vi "Transfer LLP Packets To Host.vi"(0 "tagged llp packets cluster":T1, 1 "reset":bool, 5 "end of data":bool[](array[boolean])=[FALSE, FALSE, FALSE, FALSE, FALSE, FALSE, FALSE, FALSE], 9 "tagged llp packet valid":bool[](array[boolean])=[FALSE, FALSE, FALSE, FALSE, FALSE, FALSE, FALSE, FALSE]) -> (14 "ready for input":bool[](array[boolean]))   [LabVIEW 2020, in "GettingStarted_Acq_Tap_148X_FPGA.lvlib"]
uses:
  GettingStarted_Acq_Tap_148X_FPGA.lvlib
  Common/Types/Tagged LLP Packets Cluster.ctl
  <instrlib>/FlexRIO/CSI-2/v2/FPGA/Types/Tagged LLP Packet.ctl
  <instrlib>/FlexRIO/CSI-2/v2/FPGA/Types/FPGA LLP Packet Tag.ctl
  <instrlib>/FlexRIO/CSI-2/v2/FPGA/Types/FPGA LLP Packet Timestamp.ctl
  <instrlib>/FlexRIO/CSI-2/v2/FPGA/Types/Timestamp ID.ctl
  <instrlib>/FlexRIO/CSI-2/v2/FPGA/Types/FPGA LLP Packet Size.ctl
  <instrlib>/FlexRIO/CSI-2/v2/FPGA/Types/LLP Packet.ctl
  <instrlib>/FlexRIO/CSI-2/v2/FPGA/Types/LLP Packet Header.ctl
  <instrlib>/FlexRIO/CSI-2/v2/FPGA/Types/LLP Packet Payload.ctl
  <instrlib>/FlexRIO/CSI-2/v2/FPGA/Types/LLP Packet Footer.ctl
  <instrlib>/_niInstr/Basic Elements/v1/FPGA/niInstr Basic Elements v1 FPGA.lvlib
  <instrlib>/FlexRIO/CSI-2/v2/FPGA/NI CSI-2 API FPGA v2.lvlib
  Common/GettingStarted_Common_148X_FPGA.lvlib
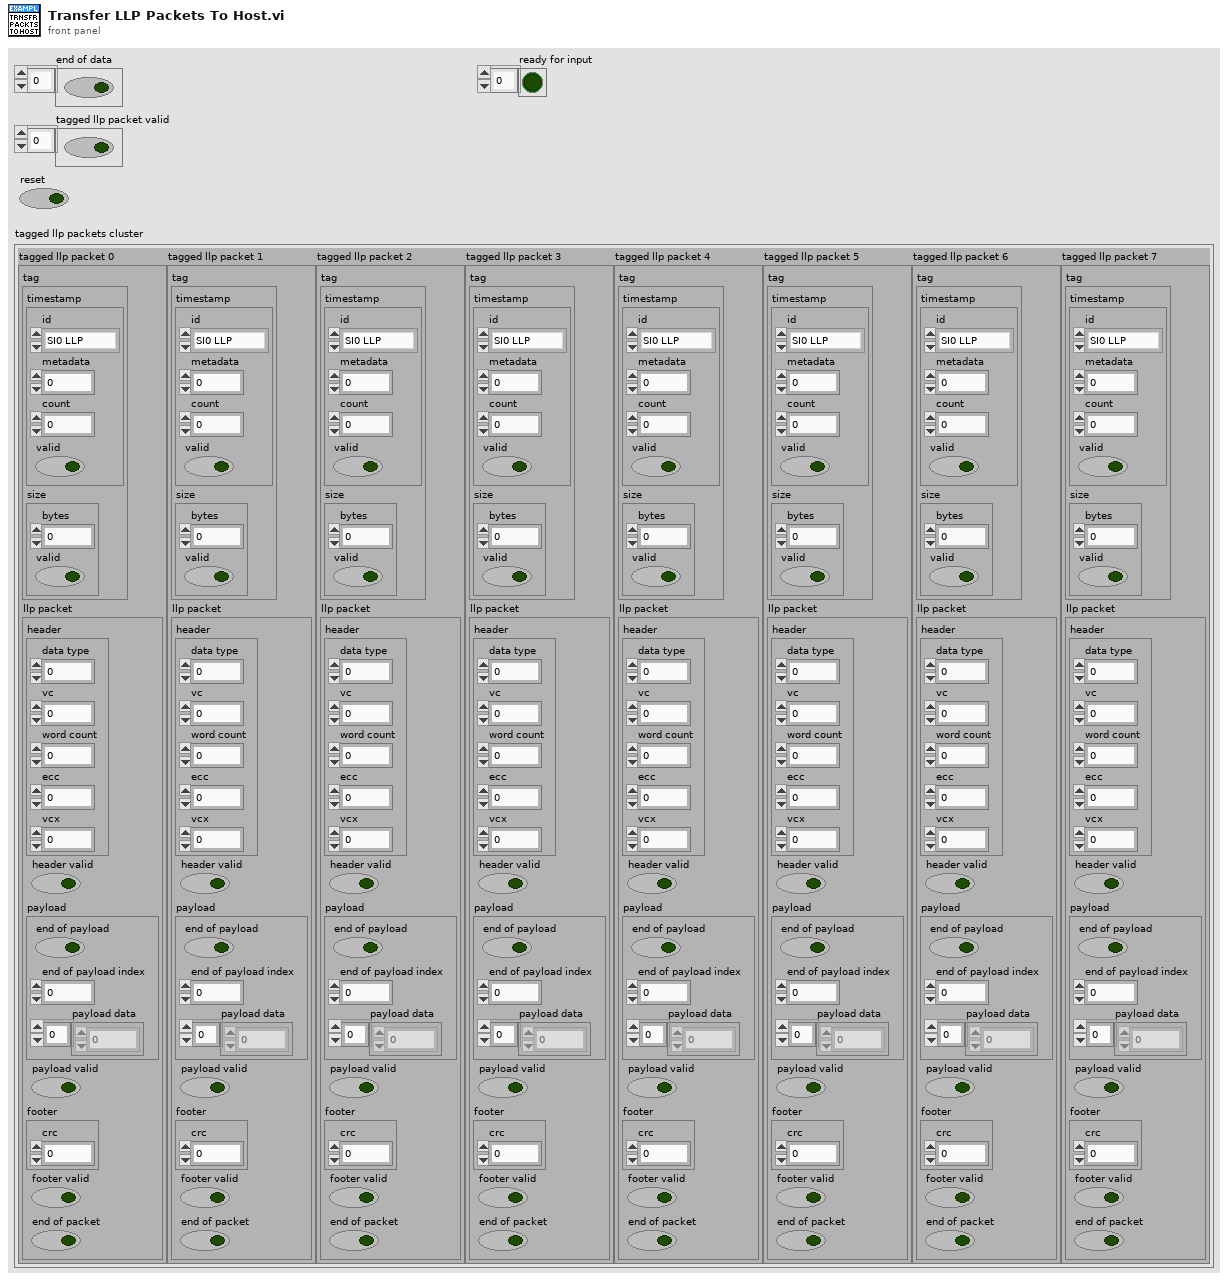
[diagram p1: front panel]
types:
  T1 = typedef "GettingStarted_Common_148X_FPGA.lvlib/Tagged LLP Packets Cluster.ctl" = cluster{"tagged llp packet 0":T2, "tagged llp packet 1":T2, "tagged llp packet 2":T2, "tagged llp packet 3":T2, "tagged llp packet 4":T2, "tagged llp packet 5":T2, "tagged llp packet 6":T2, "tagged llp packet 7":T2}
  T2 = typedef "NI CSI-2 API FPGA v2.lvlib/Tagged LLP Packet.ctl" = cluster{"tag":T3, "llp packet":T7}
  T3 = typedef "NI CSI-2 API FPGA v2.lvlib/FPGA LLP Packet Tag.ctl" = cluster{"timestamp":T4, "size":T6}
  T4 = typedef "NI CSI-2 API FPGA v2.lvlib/FPGA LLP Packet Timestamp.ctl" = cluster{"valid":bool, "count":fxp<+,50,50>, "id":T5, "metadata":u8}
  T5 = typedef "NI CSI-2 API FPGA v2.lvlib/Timestamp ID.ctl" = enum8{"SI0 LLP", "SI1 LLP", "SI2 LLP", "SI3 LLP", "SI4 LLP", "SI5 LLP", "SI6 LLP", "SI7 LLP", "SO0 LLP", "SO1 LLP", "SO2 LLP", "SO3 LLP", "SO4 LLP", "SO5 LLP", "SO6 LLP", "SO7 LLP", "Ser0 GPIO Bank", "Ser1 GPIO Bank", "Ser2 GPIO Bank", "Ser3 GPIO Bank", "Ser4 GPIO Bank", "Ser5 GPIO Bank", "Ser6 GPIO Bank", "Ser7 GPIO Bank", "Des0 GPIO Bank", "Des1 GPIO Bank", "Des2 GPIO Bank", "Des3 GPIO Bank", "Des4 GPIO Bank", "Des5 GPIO Bank", "Des6 GPIO Bank", "Des7 GPIO Bank", "User0", "User1", "User2", "User3", "User4", "User5", "User6", "User7", "User8", "User9", "User10", "User11", "User12", "User13", "User14", "User15", "User16", "User17", "User18", "User19", "User20", "User21", "User22", "User23", "User24", "User25", "User26", "User27", "User28", "User29", "User30", "User31"}
  T6 = typedef "NI CSI-2 API FPGA v2.lvlib/FPGA LLP Packet Size.ctl" = cluster{"bytes":fxp<+,17,17>, "valid":bool}
  T7 = typedef "NI CSI-2 API FPGA v2.lvlib/LLP Packet.ctl" = cluster{"header":T8, "header valid":bool, "payload":T9, "payload valid":bool, "footer":T10, "footer valid":bool, "end of packet":bool}
  T8 = typedef "NI CSI-2 API FPGA v2.lvlib/LLP Packet Header.ctl" = cluster{"word count":u16, "ecc":fxp<+,6,6>, "vcx":fxp<+,2,2>, "data type":fxp<+,6,6>, "vc":fxp<+,2,2>}
  T9 = typedef "NI CSI-2 API FPGA v2.lvlib/LLP Packet Payload.ctl" = cluster{"end of payload":bool, "end of payload index":fxp<+,3,3>, "payload data":u8[]}
  T10 = typedef "NI CSI-2 API FPGA v2.lvlib/LLP Packet Footer.ctl" = cluster{"crc":u16}
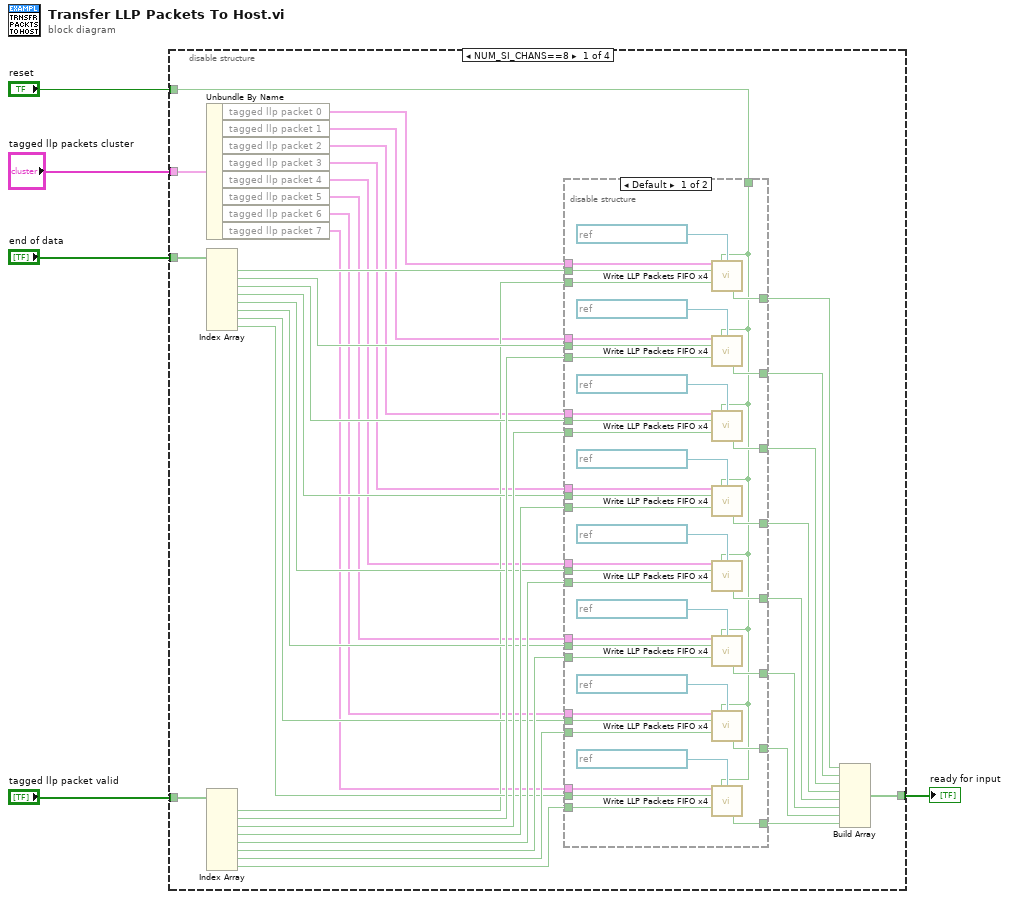
[diagram p0: block diagram]
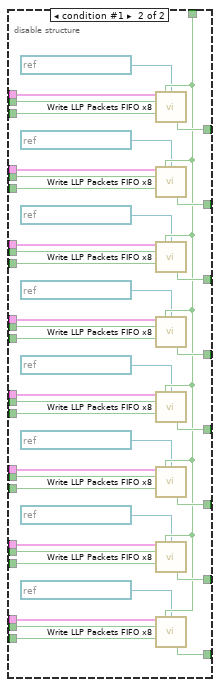
[diagram p2: hidden frame]
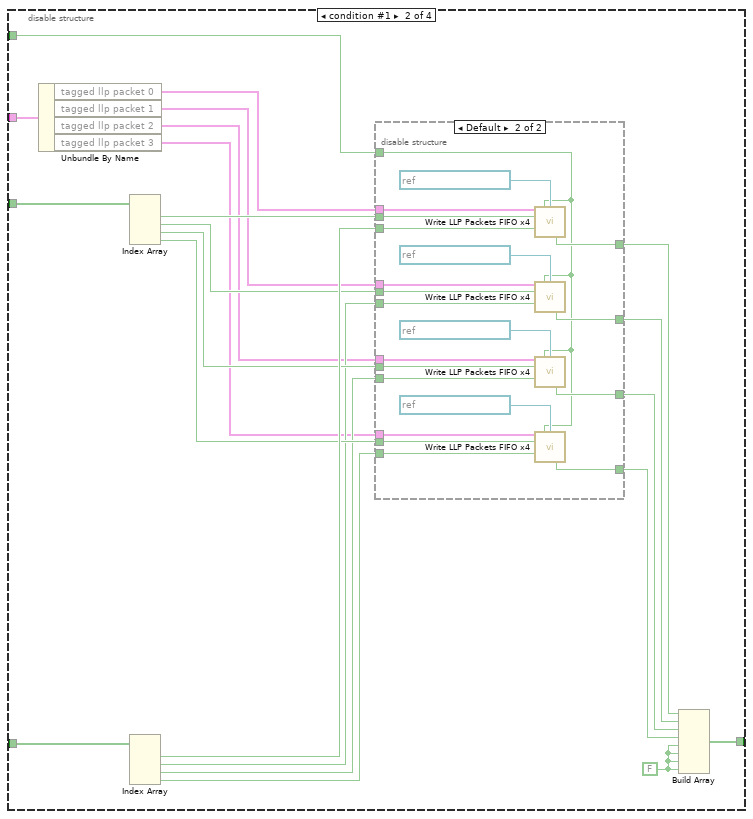
[diagram p3: hidden frame]
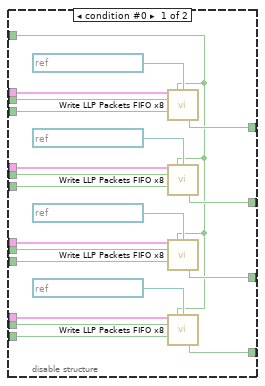
[diagram p4: hidden frame]
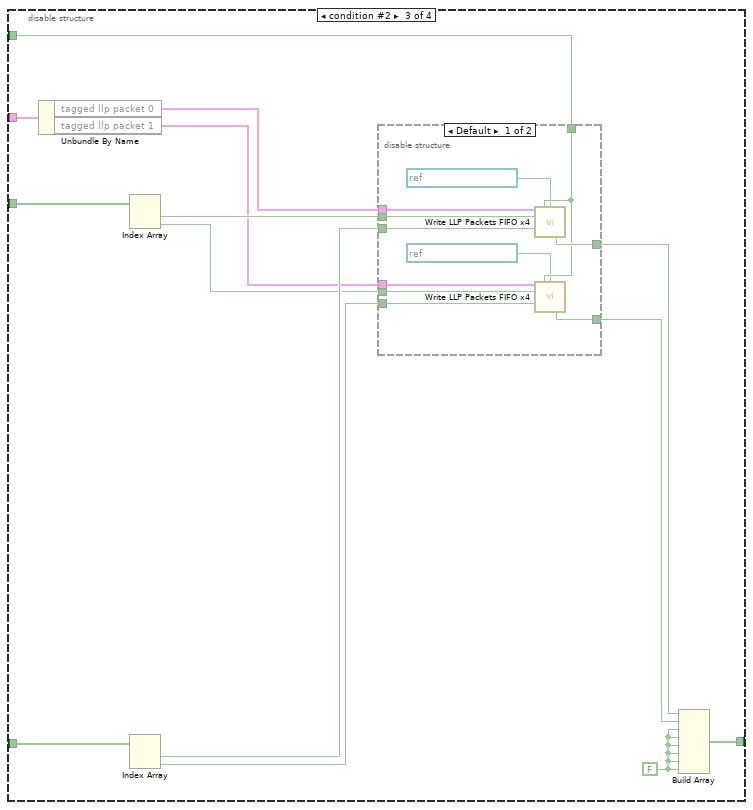
[diagram p5: hidden frame]
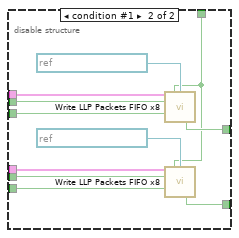
[diagram p6: hidden frame]
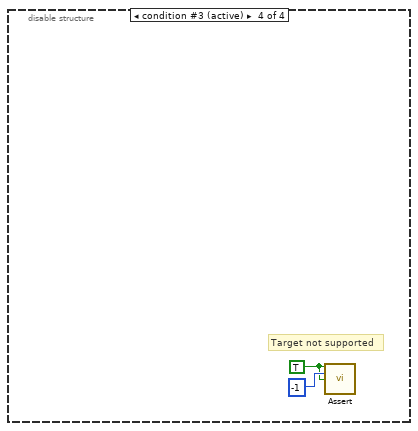
[diagram p7: hidden frame]
diagram:
  n1 = disable-structure shown="NUM_SI_CHANS==8" {
    disable-tunnel: "reset" -> [w15 w125 w193 _]
    disable-tunnel: "tagged llp packet valid" -> [w18 w133 w195 _]
    disable-tunnel: "end of data" -> [w17 w132 w194 _]
    disable-tunnel: "tagged llp packets cluster" -> [w14 w130 w192 _]
    disable-tunnel: [w16 w134 w196 _] -> w2
    frame condition #0 {
      n2 = Unbundle By Name(w14) -> ("tagged llp packet 0"=w13:T2, "tagged llp packet 1"=w6:T2, "tagged llp packet 2"=w7:T2, "tagged llp packet 3"=w8:T2, "tagged llp packet 4"=w9:T2, "tagged llp packet 5"=w10:T2, "tagged llp packet 6"=w11:T2, "tagged llp packet 7"=w12:T2)
      n3 = Index Array(array=w17) -> (element #1=w27:bool, element #2=w26:bool, element #3=w25:bool, element #4=w24:bool, element #5=w23:bool, element #6=w22:bool, element #7=w21:bool, element #8=w20:bool)  [unwired: 8 in]
      n4 = Index Array(array=w18) -> (element #1=w19:bool, element #2=w28:bool, element #3=w29:bool, element #4=w30:bool, element #5=w31:bool, element #6=w32:bool, element #7=w33:bool, element #8=w34:bool)  [unwired: 8 in]
      n5 = disable-structure shown="Default" {
        disable-tunnel: [w83 w124] -> w42
        disable-tunnel: [w82 w123] -> w41
        disable-tunnel: [w81 w122] -> w40
        disable-tunnel: [w80 w121] -> w39
        disable-tunnel: [w79 w120] -> w38
        disable-tunnel: [w78 w119] -> w37
        disable-tunnel: [w77 w118] -> w36
        disable-tunnel: [w76 w117] -> w35
        disable-tunnel: w34 -> [w75 w116]
        disable-tunnel: w33 -> [w74 w115]
        disable-tunnel: w32 -> [w73 w114]
        disable-tunnel: w31 -> [w72 w113]
        disable-tunnel: w30 -> [w71 w112]
        disable-tunnel: w29 -> [w70 w111]
        disable-tunnel: w28 -> [w69 w110]
        disable-tunnel: w27 -> [w68 w109]
        disable-tunnel: w26 -> [w67 w108]
        disable-tunnel: w25 -> [w66 w107]
        disable-tunnel: w24 -> [w65 w106]
        disable-tunnel: w23 -> [w64 w105]
        disable-tunnel: w22 -> [w63 w104]
        disable-tunnel: w21 -> [w62 w103]
        disable-tunnel: w20 -> [w61 w102]
        disable-tunnel: w19 -> [w60 w101]
        disable-tunnel: w15 -> [w51 w100]
        disable-tunnel: w13 -> [w50 w99]
        disable-tunnel: w12 -> [w49 w98]
        disable-tunnel: w11 -> [w48 w97]
        disable-tunnel: w10 -> [w47 w96]
        disable-tunnel: w9 -> [w46 w95]
        disable-tunnel: w8 -> [w45 w94]
        disable-tunnel: w7 -> [w44 w93]
        disable-tunnel: w6 -> [w43 w92]
        frame condition #0 (active) {
          n6 = call "Write LLP Packets FIFO x4.vi"("tagged llp packet"=w50, "reset"=w51, "llp packets dma fifo x4"=refnum<k21> "SI 0 LLP Packets" ("llp packets dma fifo"), "flush"=w68, "input valid"=w60) -> ("ready for input"=w83:bool)  [unwired: 10 in]
          n7 = call "Write LLP Packets FIFO x4.vi"("tagged llp packet"=w43, "reset"=w51, "llp packets dma fifo x4"=refnum<k21> "SI 1 LLP Packets" ("llp packets dma fifo"), "flush"=w67, "input valid"=w69) -> ("ready for input"=w82:bool)  [unwired: 10 in]
          n8 = call "Write LLP Packets FIFO x4.vi"("tagged llp packet"=w44, "reset"=w51, "llp packets dma fifo x4"=refnum<k21> "SI 2 LLP Packets" ("llp packets dma fifo"), "flush"=w66, "input valid"=w70) -> ("ready for input"=w81:bool)  [unwired: 10 in]
          n9 = call "Write LLP Packets FIFO x4.vi"("tagged llp packet"=w45, "reset"=w51, "llp packets dma fifo x4"=refnum<k21> "SI 3 LLP Packets" ("llp packets dma fifo"), "flush"=w65, "input valid"=w71) -> ("ready for input"=w80:bool)  [unwired: 10 in]
          n10 = call "Write LLP Packets FIFO x4.vi"("tagged llp packet"=w46, "reset"=w51, "llp packets dma fifo x4"=refnum<k21> "SI 4 LLP Packets" ("llp packets dma fifo"), "flush"=w64, "input valid"=w72) -> ("ready for input"=w79:bool)  [unwired: 10 in]
          n11 = call "Write LLP Packets FIFO x4.vi"("tagged llp packet"=w47, "reset"=w51, "llp packets dma fifo x4"=refnum<k21> "SI 5 LLP Packets" ("llp packets dma fifo"), "flush"=w63, "input valid"=w73) -> ("ready for input"=w78:bool)  [unwired: 10 in]
          n12 = call "Write LLP Packets FIFO x4.vi"("tagged llp packet"=w48, "reset"=w51, "llp packets dma fifo x4"=refnum<k21> "SI 6 LLP Packets" ("llp packets dma fifo"), "flush"=w62, "input valid"=w74) -> ("ready for input"=w77:bool)  [unwired: 10 in]
          n13 = call "Write LLP Packets FIFO x4.vi"("tagged llp packet"=w49, "reset"=w51, "llp packets dma fifo x4"=refnum<k21> "SI 7 LLP Packets" ("llp packets dma fifo"), "flush"=w61, "input valid"=w75) -> ("ready for input"=w76:bool)  [unwired: 10 in]
        }
        frame condition #1 {
          n14 = call "Write LLP Packets FIFO x8.vi"("tagged llp packet"=w99, "reset"=w100, "llp packets dma fifo x8"=refnum<k21> "SI 0 LLP Packets" ("llp packets dma fifo"), "flush"=w109, "input valid"=w101) -> ("ready for input"=w124:bool)  [unwired: 10 in]
          n15 = call "Write LLP Packets FIFO x8.vi"("tagged llp packet"=w92, "reset"=w100, "llp packets dma fifo x8"=refnum<k21> "SI 1 LLP Packets" ("llp packets dma fifo"), "flush"=w108, "input valid"=w110) -> ("ready for input"=w123:bool)  [unwired: 10 in]
          n16 = call "Write LLP Packets FIFO x8.vi"("tagged llp packet"=w93, "reset"=w100, "llp packets dma fifo x8"=refnum<k21> "SI 2 LLP Packets" ("llp packets dma fifo"), "flush"=w107, "input valid"=w111) -> ("ready for input"=w122:bool)  [unwired: 10 in]
          n17 = call "Write LLP Packets FIFO x8.vi"("tagged llp packet"=w94, "reset"=w100, "llp packets dma fifo x8"=refnum<k21> "SI 3 LLP Packets" ("llp packets dma fifo"), "flush"=w106, "input valid"=w112) -> ("ready for input"=w121:bool)  [unwired: 10 in]
          n18 = call "Write LLP Packets FIFO x8.vi"("tagged llp packet"=w95, "reset"=w100, "llp packets dma fifo x8"=refnum<k21> "SI 4 LLP Packets" ("llp packets dma fifo"), "flush"=w105, "input valid"=w113) -> ("ready for input"=w120:bool)  [unwired: 10 in]
          n19 = call "Write LLP Packets FIFO x8.vi"("tagged llp packet"=w96, "reset"=w100, "llp packets dma fifo x8"=refnum<k21> "SI 5 LLP Packets" ("llp packets dma fifo"), "flush"=w104, "input valid"=w114) -> ("ready for input"=w119:bool)  [unwired: 10 in]
          n20 = call "Write LLP Packets FIFO x8.vi"("tagged llp packet"=w97, "reset"=w100, "llp packets dma fifo x8"=refnum<k21> "SI 6 LLP Packets" ("llp packets dma fifo"), "flush"=w103, "input valid"=w115) -> ("ready for input"=w118:bool)  [unwired: 10 in]
          n21 = call "Write LLP Packets FIFO x8.vi"("tagged llp packet"=w98, "reset"=w100, "llp packets dma fifo x8"=refnum<k21> "SI 7 LLP Packets" ("llp packets dma fifo"), "flush"=w102, "input valid"=w116) -> ("ready for input"=w117:bool)  [unwired: 10 in]
        }
      }
      n22 = Build Array(w42, w41, w40, w39, w38, w37, w36, w35) -> (w16:bool[])
    }
    frame condition #1 {
      w131 = FALSE ("element")
      n23 = Unbundle By Name(w130) -> ("tagged llp packet 0"=w129:T2, "tagged llp packet 1"=w128:T2, "tagged llp packet 2"=w127:T2, "tagged llp packet 3"=w126:T2)
      n24 = Index Array(array=w132) -> (element #1=w142:bool, element #2=w143:bool, element #3=w144:bool, element #4=w145:bool)  [unwired: 4 in]
      n25 = Index Array(array=w133) -> (element #1=w146:bool, element #2=w141:bool, element #3=w140:bool, element #4=w139:bool)  [unwired: 4 in]
      n26 = disable-structure shown="Default" {
        disable-tunnel: w146 -> [w167 w188]
        disable-tunnel: w145 -> [w166 w187]
        disable-tunnel: w144 -> [w165 w186]
        disable-tunnel: w143 -> [w164 w185]
        disable-tunnel: w142 -> [w163 w184]
        disable-tunnel: w141 -> [w162 w183]
        disable-tunnel: w140 -> [w161 w182]
        disable-tunnel: w139 -> [w160 w181]
        disable-tunnel: [w159 w180] -> w138
        disable-tunnel: [w158 w179] -> w137
        disable-tunnel: [w157 w178] -> w136
        disable-tunnel: [w156 w177] -> w135
        disable-tunnel: w129 -> [w151 w172]
        disable-tunnel: w128 -> [w150 w171]
        disable-tunnel: w127 -> [w149 w170]
        disable-tunnel: w126 -> [w148 w169]
        disable-tunnel: w125 -> [w147 w168]
        frame condition #0 {
          n27 = call "Write LLP Packets FIFO x8.vi"("tagged llp packet"=w151, "reset"=w147, "llp packets dma fifo x8"=refnum<k21> "SI 0 LLP Packets" ("llp packets dma fifo"), "flush"=w163, "input valid"=w167) -> ("ready for input"=w156:bool)  [unwired: 10 in]
          n28 = call "Write LLP Packets FIFO x8.vi"("tagged llp packet"=w150, "reset"=w147, "llp packets dma fifo x8"=refnum<k21> "SI 1 LLP Packets" ("llp packets dma fifo"), "flush"=w164, "input valid"=w162) -> ("ready for input"=w157:bool)  [unwired: 10 in]
          n29 = call "Write LLP Packets FIFO x8.vi"("tagged llp packet"=w149, "reset"=w147, "llp packets dma fifo x8"=refnum<k21> "SI 2 LLP Packets" ("llp packets dma fifo"), "flush"=w165, "input valid"=w161) -> ("ready for input"=w158:bool)  [unwired: 10 in]
          n30 = call "Write LLP Packets FIFO x8.vi"("tagged llp packet"=w148, "reset"=w147, "llp packets dma fifo x8"=refnum<k21> "SI 3 LLP Packets" ("llp packets dma fifo"), "flush"=w166, "input valid"=w160) -> ("ready for input"=w159:bool)  [unwired: 10 in]
        }
        frame condition #1 (active) {
          n31 = call "Write LLP Packets FIFO x4.vi"("tagged llp packet"=w172, "reset"=w168, "llp packets dma fifo x4"=refnum<k21> "SI 0 LLP Packets" ("llp packets dma fifo"), "flush"=w184, "input valid"=w188) -> ("ready for input"=w177:bool)  [unwired: 10 in]
          n32 = call "Write LLP Packets FIFO x4.vi"("tagged llp packet"=w171, "reset"=w168, "llp packets dma fifo x4"=refnum<k21> "SI 1 LLP Packets" ("llp packets dma fifo"), "flush"=w185, "input valid"=w183) -> ("ready for input"=w178:bool)  [unwired: 10 in]
          n33 = call "Write LLP Packets FIFO x4.vi"("tagged llp packet"=w170, "reset"=w168, "llp packets dma fifo x4"=refnum<k21> "SI 2 LLP Packets" ("llp packets dma fifo"), "flush"=w186, "input valid"=w182) -> ("ready for input"=w179:bool)  [unwired: 10 in]
          n34 = call "Write LLP Packets FIFO x4.vi"("tagged llp packet"=w169, "reset"=w168, "llp packets dma fifo x4"=refnum<k21> "SI 3 LLP Packets" ("llp packets dma fifo"), "flush"=w187, "input valid"=w181) -> ("ready for input"=w180:bool)  [unwired: 10 in]
        }
      }
      n35 = Build Array(w135, w136, w137, w138, w131, w131, w131, w131) -> (w134:bool[])
    }
    frame condition #2 {
      w189 = FALSE ("element")
      n36 = Unbundle By Name(w192) -> ("tagged llp packet 0"=w191:T2, "tagged llp packet 1"=w190:T2)
      n37 = Index Array(array=w194) -> (element #1=w200:bool, element #2=w201:bool)  [unwired: 2 in]
      n38 = Index Array(array=w195) -> (element #1=w202:bool, element #2=w199:bool)  [unwired: 2 in]
      n39 = disable-structure shown="Default" {
        disable-tunnel: w202 -> [w213 w224]
        disable-tunnel: w201 -> [w212 w223]
        disable-tunnel: w200 -> [w211 w222]
        disable-tunnel: w199 -> [w210 w221]
        disable-tunnel: [w209 w220] -> w198
        disable-tunnel: [w208 w219] -> w197
        disable-tunnel: w193 -> [w207 w216]
        disable-tunnel: w191 -> [w206 w215]
        disable-tunnel: w190 -> [w205 w214]
        frame condition #0 (active) {
          n40 = call "Write LLP Packets FIFO x4.vi"("tagged llp packet"=w206, "reset"=w207, "llp packets dma fifo x4"=refnum<k21> "SI 0 LLP Packets" ("llp packets dma fifo"), "flush"=w211, "input valid"=w213) -> ("ready for input"=w208:bool)  [unwired: 10 in]
          n41 = call "Write LLP Packets FIFO x4.vi"("tagged llp packet"=w205, "reset"=w207, "llp packets dma fifo x4"=refnum<k21> "SI 1 LLP Packets" ("llp packets dma fifo"), "flush"=w212, "input valid"=w210) -> ("ready for input"=w209:bool)  [unwired: 10 in]
        }
        frame condition #1 {
          n42 = call "Write LLP Packets FIFO x8.vi"("tagged llp packet"=w215, "reset"=w216, "llp packets dma fifo x8"=refnum<k21> "SI 0 LLP Packets" ("llp packets dma fifo"), "flush"=w222, "input valid"=w224) -> ("ready for input"=w219:bool)  [unwired: 10 in]
          n43 = call "Write LLP Packets FIFO x8.vi"("tagged llp packet"=w214, "reset"=w216, "llp packets dma fifo x8"=refnum<k21> "SI 1 LLP Packets" ("llp packets dma fifo"), "flush"=w223, "input valid"=w221) -> ("ready for input"=w220:bool)  [unwired: 10 in]
        }
      }
      n44 = Build Array(w197, w198, w189, w189, w189, w189, w189, w189) -> (w196:bool[])
    }
    frame condition #3 (active) {
      w225 = TRUE ("assert")
      # "Target not supported"
      n45 = call <instrlib>:"Assert.vi"("assert"=w225, "error code"=-1, "enable show error"=w225) -> ()  [unwired: 13 in]
    }
  }
  "ready for input" <- w2
